vi "Extract Single Pixel Velocity(SubVI).vi"(6 "Velocity Component 2":T1, 8 "limit":sgl, 9 "Rectangle":cluster{dbl, dbl, dbl, dbl, dbl}, 11 "Velocity Component 1":T1) -> (2 "Vector sum Comp 2":dbl, 3 "Vector sum Comp 1":dbl)   [LabVIEW 2014]
uses:
  <vilib>/vision/Image Controls.llb/IMAQ Image.ctl
  <vilib>/Analysis/baseanly.llb/Normalize Matrix.vi
  <vilib>/Analysis/NI_AALBase.lvlib
panel:
  out "mean 2":dbl(slide) scale=-10.0..10.0
  out "mean 1":dbl(slide) scale=-10.0..10.0
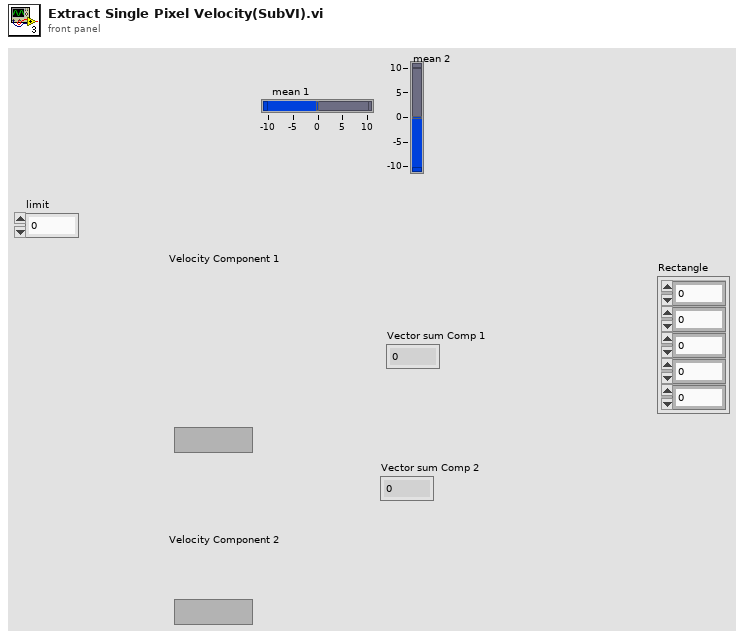
[diagram p1: front panel]
types:
  T1 = typedef "IMAQ Image.ctl" = refnum<image>
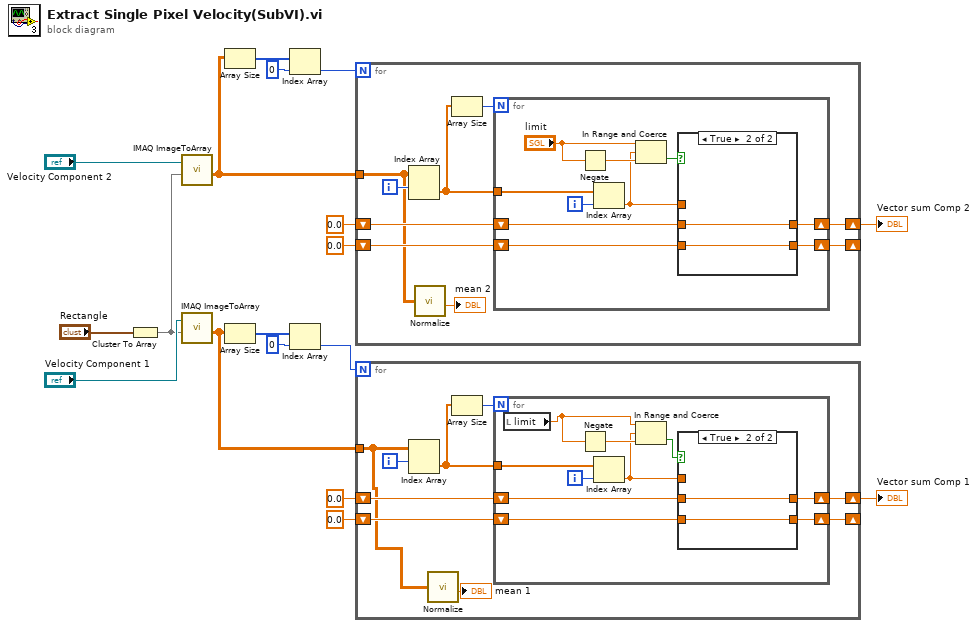
[diagram p0: block diagram]
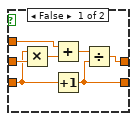
[diagram p2: hidden frame]
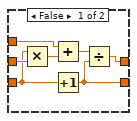
[diagram p3: hidden frame]
diagram:
  n1 = Cluster To Array(cluster="Rectangle") -> (array=w15:dbl[])
  n2 = call "IMAQ ImageToArray"("Optional Rectangle"=w15, "Image"="Velocity Component 2") -> ("Image Pixels (Float)"=w9:sgl[][])  [unwired: 2 in, 4 out]
  n3 = call "IMAQ ImageToArray"("Optional Rectangle"=w15, "Image"="Velocity Component 1") -> ("Image Pixels (Float)"=w2:sgl[][])  [unwired: 2 in, 4 out]
  n4 = Array Size(array=w9) -> (size(s)=w12:i32[])
  n5 = Array Size(array=w2) -> (size(s)=w14:i32[])
  n6 = Index Array(array=w12, index=0) -> (element=w8:i32)
  n7 = Index Array(array=w14, index=0) -> (element=w3:i32)
  n8 = for {
    N: w8 -> [_]
    tunnel: w9 -> [w20]
    shift-right: [w23] -> w7
    shift-left: 0.0 -> [w25]
    shift-right: [w21] -> _
    shift-left: 0.0 -> [w22]
    i -> [w27]
    n9 = Index Array(array=w20, index (row)=w27) -> (element=w26:sgl[])  [unwired: 1 in]
    n10 = call-poly <vilib>:"Normalize.vi"("Matrix"=w20) -> ("mean"=→"mean 2":dbl)  [unwired: 1 in, 3 out]
    n11 = Array Size(array=w26) -> (size(s)=w24:i32)
    n12 = for {
      N: w24 -> [_]
      tunnel: w26 -> [w37]
      shift-right: [w30] -> w23
      shift-left: w25 -> [w31]
      shift-right: [w28] -> w21
      shift-left: w22 -> [w29]
      i -> [w36]
      n13 = Negate(x="limit") -> (-x=w35:sgl)
      n14 = Index Array(array=w37, index=w36) -> (element=w32:sgl)
      n15 = In Range and Coerce(upper limit="limit", x=w32, lower limit=w35) -> (In Range?=w33:bool)  [unwired: 1 out]
      n16 = case shown="True" w33 {
        tunnel: w32 -> [w42 _]
        tunnel: w31 -> [w44 w45]
        tunnel: [w40 w45] -> w30
        tunnel: w29 -> [w39 w46]
        tunnel: [w38 w46] -> w28
        frame False {
          n17 = Multiply(x=w39, y=w44) -> (x*y=w43:dbl)
          n18 = Add(x=w42, y=w43) -> (x+y=w41:dbl)
          n19 = Increment(x=w39) -> (x+1=w38:dbl)
          n20 = Divide(x=w41, y=w38) -> (x/y=w40:dbl)
        }
        frame True {
        }
      }
    }
  }
  "Vector sum Comp 2" <- w7
  n21 = for {
    N: w3 -> [_]
    tunnel: w2 -> [w48]
    shift-right: [w51] -> w1
    shift-left: 0.0 -> [w53]
    shift-right: [w49] -> _
    shift-left: 0.0 -> [w50]
    i -> [w55]
    n22 = Index Array(array=w48, index (row)=w55) -> (element=w54:sgl[])  [unwired: 1 in]
    n23 = call-poly <vilib>:"Normalize.vi"("Matrix"=w48) -> ("mean"=→"mean 1":dbl)  [unwired: 1 in, 3 out]
    n24 = Array Size(array=w54) -> (size(s)=w52:i32)
    n25 = for {
      N: w52 -> [_]
      tunnel: w54 -> [w56]
      shift-right: [w60] -> w51
      shift-left: w53 -> [w61]
      shift-right: [w58] -> w49
      shift-left: w50 -> [w59]
      i -> [w65]
      n26 = local read "limit"() -> (w57:sgl)
      n27 = Negate(x=w57) -> (-x=w64:sgl)
      n28 = Index Array(array=w56, index=w65) -> (element=w62:sgl)
      n29 = In Range and Coerce(upper limit=w57, x=w62, lower limit=w64) -> (In Range?=w63:bool)  [unwired: 1 out]
      n30 = case shown="True" w63 {
        tunnel: w62 -> [w70 _]
        tunnel: w61 -> [w72 w73]
        tunnel: [w68 w73] -> w60
        tunnel: w59 -> [w67 w74]
        tunnel: [w66 w74] -> w58
        frame False {
          n31 = Multiply(x=w67, y=w72) -> (x*y=w71:dbl)
          n32 = Add(x=w70, y=w71) -> (x+y=w69:dbl)
          n33 = Increment(x=w67) -> (x+1=w66:dbl)
          n34 = Divide(x=w69, y=w66) -> (x/y=w68:dbl)
        }
        frame True {
        }
      }
    }
  }
  "Vector sum Comp 1" <- w1
